vi "Get COM Port Name.vi"() -> ()   [LabVIEW 2011]
panel:
  out "Array":string[](array[string])
  out "find list":string[](array[string])
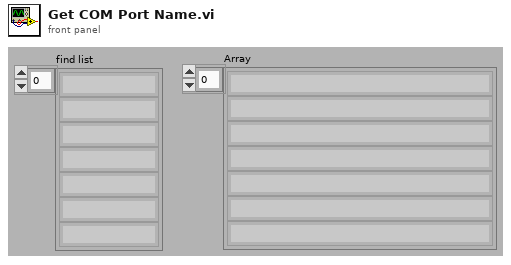
[diagram p1: front panel]
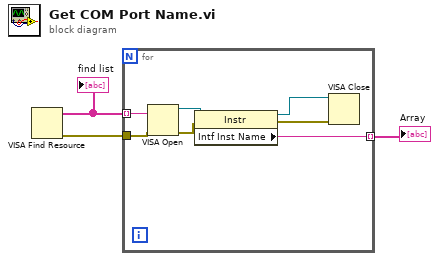
[diagram p0: block diagram]
diagram:
  n1 = VISA Find Resource() -> (0:w3:errorcluster, 3:w2:string[])  [unwired: 3 in, 1 out]
  "find list" <- w2
  n2 = for {
    tunnel: w2 -> [w8] mode=indexing
    tunnel: [w7] -> w1 mode=indexing
    tunnel: w3 -> [w4]
    n3 = VISA Open(error in (no error)=w4, VISA resource name=w8) -> (VISA resource name=w10:refnum<visa-resource-name>, error out=w9:errorcluster)  [unwired: 3 in]
    n4 = property class="Instr"(reference=w10, error in=w9) -> (reference out=w6:refnum<visa-resource-name>, error out=w5:errorcluster, "Intf Inst Name"=w7:string)
    n5 = VISA Close(VISA resource name=w6, error in (no error)=w5) -> ()  [unwired: 1 out]
  }
  "Array" <- w1
